vi "Startup_Instrument_Selection.vi"() -> ()   [LabVIEW 2014]
uses:
  <vilib>/Platform/TimedLoop/XDataNode/timing_clust.ctl
  <vilib>/Platform/TimedLoop/XDataNode/nitl_modes.ctl
  <vilib>/Platform/TimedLoop/XDataNode/wakeup.ctl
  <vilib>/Instr/_visa.llb/VISA Set IO Buffer Mask.ctl
  <vilib>/Instr/_visa.llb/VISA Configure Serial Port (Instr).vi
  <vilib>/platform/TimedLoop/XDataNode/XDataNode.xnode
  <vilib>/Platform/TimedLoop/XDataNode/XDNodeRunTimeDep.lvlib
panel:
  in  "Ozone_TEi_49i_ID":string="»"
  in  "SO2_TEi_43i_ID":string="µ"
  in  "SO2_TEi_43c_ID":string="«"
  in  "Ozone_TEi_49c_ID":string="±"
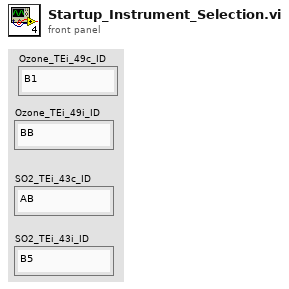
[diagram p1: front panel]
types:
  T1 = typedef "XDNodeRunTimeDep.lvlib/timing_clust.ctl" = cluster{"Expected End [f-1]":u64, "Actual End [f-1]":u64, "Finished Late? [f-1]":bool, "Expected End [i-1]":u64, "Actual End [i-1]":u64, "Finished Late? [i-1]":bool, "Expected Start [i]":u64, "Actual Start [i]":u64, "Expected Start [f]":u64, "Actual Start [f]":u64, "Source Name":string, "Structure Name":string, "Period":i64, "Deadline":i64, "Offset":i64, "Start":i64, "Priority":i32, "Timeout":i32, "Mode":T2, "Wakeup Reason":T3, "Error":errorcluster, "Source Type":string, "Secondary Source Type":string, "Global End Time":u64, "Global Start Time":u64, "Frame Duration":u64, "Iteration Duration":u64, "Assigned CPU":i32, "I/O Scan Engine Mode":u32}
  T2 = typedef "XDNodeRunTimeDep.lvlib/nitl_modes.ctl" = enum32{"No Change", "Process missed periods, maintain original phase", "Discard missed periods, maintain original phase", "Process missed periods, ignore original phase", "Discard missed periods, ignore original phase"}
  T3 = typedef "XDNodeRunTimeDep.lvlib/wakeup.ctl" = enum32{"Normal", "Aborted", "Asynchronous wakeup", "Timing source error", "Timed loop error", "Timeout"}
  T4 = typedef "VISA Set IO Buffer Mask.ctl" = u16
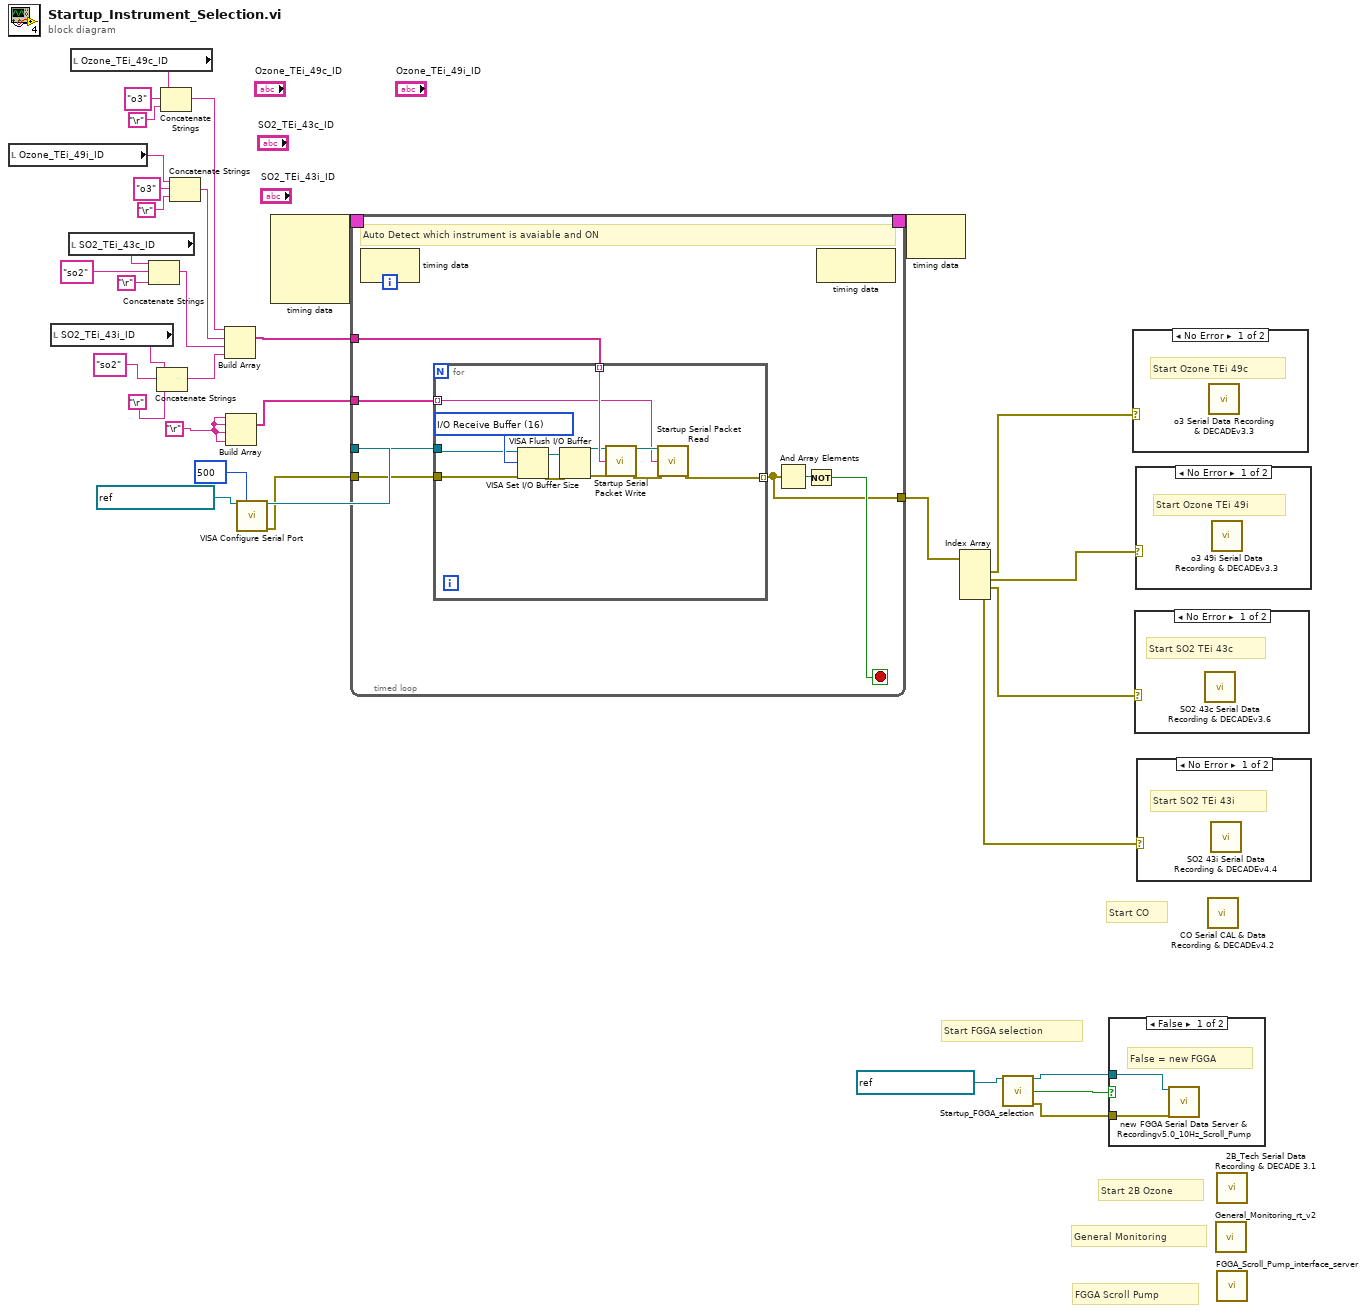
[diagram p0: block diagram]
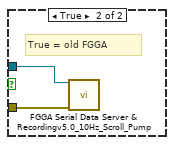
[diagram p6: hidden frame]
diagram:
  w5 = "\r"
  # "FGGA Scroll Pump"
  # "Start 2B Ozone"
  # "Start CO"
  # "General Monitoring"
  # "Start FGGA selection"
  n1 = local read "Ozone_TEi_49i_ID"() -> (w10:string)
  n2 = local read "SO2_TEi_43i_ID"() -> (w20:string)
  n3 = local read "SO2_TEi_43c_ID"() -> (w27:string)
  n4 = local read "Ozone_TEi_49c_ID"() -> (w23:string)
  n5 = Concatenate Strings(w27, "so2" ("string"), "\r") -> (w13:string)
  n6 = Concatenate Strings(w20, "so2" ("string"), "\r") -> (w14:string)
  n7 = Concatenate Strings(w23, "o3" ("string"), "\r") -> (w19:string)
  n8 = Concatenate Strings(w10, "o3" ("string"), "\r") -> (w9:string)
  n9 = Build Array(w19, w9, w13, w14) -> (w18:string[])
  n10 = Build Array(w5, w5, w5, w5) -> (w17:string[])
  n11 = call-poly "VISA Configure Serial Port"("VISA resource name"=refnum<visa-resource-name> "ASRL6::INSTR", "timeout (10sec)"=u32 500) -> ("VISA resource name out"=w31:refnum<visa-resource-name>, "error out"=w30:errorcluster)  [unwired: 12 in]
  n12 = node-c288() -> (w34:T1)  [unwired: 4 in]
  n13 = timed-loop {
    tunnel: w31 -> [w41]
    tunnel: w30 -> [w40]
    timing: w34 -> [_]
    timing-out: [_] -> w33
    tunnel: w18 -> [w39]
    tunnel: w17 -> [w38]
    tunnel: [w35] -> w16
    stop <- w36 stop-if-true
    # "Auto Detect which instrument is avaiable and ON"
    n14 = node-c288() -> ()  [unwired: 1 in, 1 out]
    n15 = for {
      tunnel: w41 -> [w45]
      tunnel: w40 -> [w44]
      tunnel: w39 -> [w51] mode=indexing
      tunnel: w38 -> [w50] mode=indexing
      tunnel: [w49] -> w35 mode=indexing
      w46 = T4 16 items=["I/O Receive Buffer"=16, "I/O Transmit Buffer"=32, "I/O Receive and Transmit Buffer"=48] ("Mask")
      n16 = VISA Set I/O Buffer Size(VISA resource name=w45, mask (16)=w46, error in (no error)=w44) -> (VISA resource name out=w47:refnum<visa-resource-name>, error out=w48:errorcluster)  [unwired: 1 in]
      n17 = VISA Flush I/O Buffer(VISA resource name=w47, error in (no error)=w48) -> (VISA resource name out=w42:refnum<visa-resource-name>, error out=w43:errorcluster)  [unwired: 1 in]
      n18 = call "Startup Serial Packet Write.vi"("VISA resource name In"=w42, "Data in"=w51, "error in (no error)"=w43) -> ("VISA resource name Out"=w52:refnum<visa-resource-name>, "error out"=w53:errorcluster)  [unwired: 11 in]
      n19 = call "Startup Serial Packet Read.vi"("VISA resource In"=w52, "End Character"=w50, "error in"=w53) -> ("error out"=w49:errorcluster)  [unwired: 10 in, 2 out]
    }
    n20 = And Array Elements(Boolean array=w35) -> (logical AND=w37:bool)
    n21 = Not(x=w37) -> (.not. x?=w36:bool)
    n22 = node-c288() -> ()  [unwired: 1 in, 1 out]
  }
  n23 = node-c288(w33) -> ()  [unwired: 1 out]
  n24 = Index Array(array=w16) -> (element #1=w15:errorcluster, element #2=w6:errorcluster, element #3=w8:errorcluster, element #4=w7:errorcluster)  [unwired: 4 in]
  n25 = call "Startup_FGGA_selection.vi"("VISA resource name"=refnum<visa-resource-name> "ASRL7::INSTR") -> ("VISA resource name out"=w3:refnum<visa-resource-name>, "old FGGA = True\nnew FGGA = False"=w2:bool, "error out"=w1:errorcluster)  [unwired: 12 in]
  n26 = case shown="False" w2 {
    tunnel: w3 -> [w57 w59]
    tunnel: w1 -> [w56 w58]
    frame False {
      # "False = new FGGA"
      n27 = call "new FGGA Serial Data Server & Recordingv5.0_10Hz_Scroll_Pump.vi"("VISA resource name out"=w57, "error IO"=w56) -> ()  [unwired: 14 in]
    }
    frame True {
      # "True = old FGGA"
      n28 = call "FGGA Serial Data Server & Recordingv5.0_10Hz_Scroll_Pump.vi"("VISA resource name out"=w59, "error IO"=w58) -> ()  [unwired: 14 in]
    }
  }
  n29 = case shown="No Error" w15 {
    frame No Error {
      # "Start Ozone TEi 49c"
      n30 = call "o3 Serial Data Recording & DECADEv3.3.vi"() -> ()  [unwired: 12 in]
    }
    frame Error {
    }
  }
  n31 = case shown="No Error" w8 {
    frame No Error {
      # "Start SO2 TEi 43c"
      n32 = call "SO2 43c Serial Data Recording & DECADEv3.6.vi"() -> ()  [unwired: 12 in]
    }
    frame Error {
    }
  }
  n33 = case shown="No Error" w6 {
    frame No Error {
      # "Start Ozone TEi 49i"
      n34 = call "o3 49i Serial Data Recording & DECADEv3.3.vi"() -> ()  [unwired: 12 in]
    }
    frame Error {
    }
  }
  n35 = case shown="No Error" w7 {
    frame No Error {
      # "Start SO2 TEi 43i"
      n36 = call "SO2 43i Serial Data Recording & DECADEv4.4.vi"() -> ()  [unwired: 12 in]
    }
    frame Error {
    }
  }
  n37 = call "CO Serial CAL & Data Recording & DECADEv4.2.vi"() -> ()  [unwired: 12 in]
  n38 = call "General_Monitoring_rt_v2.vi"() -> ()  [unwired: 12 in]
  n39 = call "2B_Tech Serial Data Recording & DECADE 3.1.vi"() -> ()  [unwired: 12 in]
  n40 = call "FGGA_Scroll_Pump_interface_server.vi"() -> ()  [unwired: 12 in]
